vi "Sequence.GetiStepProperties.vi"(7 "Iteration":string, 8 "error in (no error)":errorcluster, 11 "Elements":T1[](array[typedef])) -> (0 "error out":errorcluster, 1 "Step Conatins iStep?":bool, 3 "iStepForLoop Ref":refnum<k24>)   [LabVIEW 2013, in "Simple Sequence Tools - Editor.lvlib"]
uses:
  Simple Sequence Tools - Editor.lvlib
  Types/Compiled.StepElementProperties.ctl
  Shared/Types/Channel.Properties.ctl
  Shared/Types/Step.Types.ctl
  NationalInstruments.VeriStand.RealTimeSequenceDefinitionApi
  Shared/SubVIs/Main.Constants.vi
  Shared/Simple Sequence Tools - Shared.lvlib
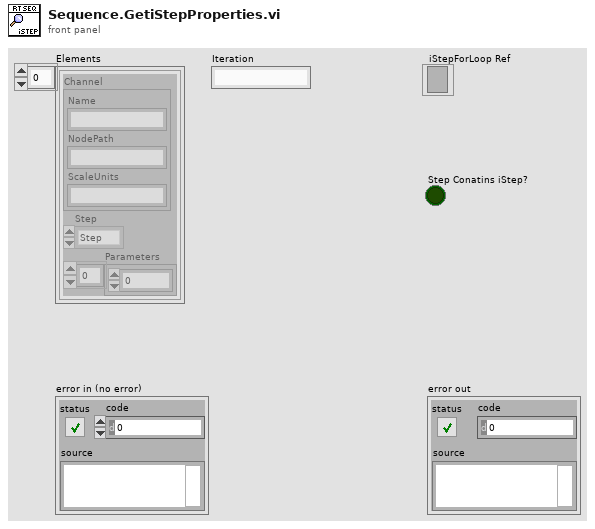
[diagram p1: front panel]
types:
  T1 = typedef "Simple Sequence Tools - Editor.lvlib/Compiled.StepElementProperties.ctl" = cluster{"Channel":T2, "Step":T3, "Parameters":dbl[]}
  T2 = typedef "Simple Sequence Tools - Shared.lvlib/Channel.Properties.ctl" = cluster{"Name":string, "NodePath":string, "ScaleUnits":string}
  T3 = typedef "Simple Sequence Tools - Shared.lvlib/Step.Types.ctl" = enum8{"Step", "iStep", "Ramp", "Unchanged", "Unknown", "Sine", "LogSine", "LinearSine", "ForcedRamp"}
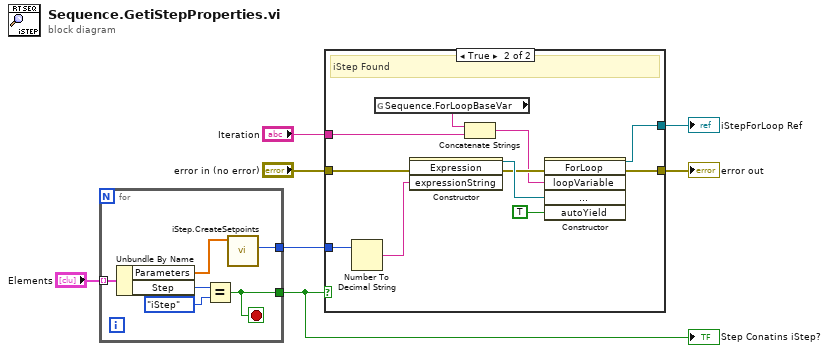
[diagram p0: block diagram]
diagram:
  n1 = for {
    tunnel: "Elements" -> [w13] mode=indexing
    tunnel: [w8] -> w5
    tunnel: [w10] -> w3
    stop <- w10 stop-if-true
    n2 = Unbundle By Name(w13) -> ("Parameters"=w9:dbl[], "Step"=w12:T3)
    n3 = Equal?(x=w12, y=Step.Types."iStep") -> (x = y?=w10:bool)
    n4 = call "iStep.CreateSetpoints.vi"("Parameters"=w9) -> ("samples"=w8:i32)  [unwired: 9 in, 1 out]
  }
  "Step Conatins iStep?" <- w3
  n5 = case shown="True" w3 {
    tunnel: "error in (no error)" -> [w14 w23]
    tunnel: [w14 w22] -> w6
    tunnel: w5 -> [_ w21]
    tunnel: [_ w19] -> w4
    tunnel: "Iteration" -> [_ w17]
    frame False {
      # "No iStep in step"
    }
    frame True {
      # "iStep Found"
      n6 = Number To Decimal String(number=w21) -> (decimal integer string=w20:string)  [unwired: 1 in]
      n7 = global read "Main.Constants.vi" "Sequence.ForLoopBaseVar"() -> (w15:string)
      n8 = constructor class="Expression"(error in=w23, "expressionString"=w20) -> (reference out=w25:refnum<k24>, error out=w24:errorcluster)  [unwired: 2 in, 2 out]
      n9 = Concatenate Strings(w15, w17) -> (w16:string)
      n10 = constructor class="ForLoop"(error in=w24, "loopVariable"=w16, "iterations"=w25, "autoYield"=TRUE) -> (reference out=w19:refnum<k24>, error out=w22:errorcluster)  [unwired: 2 in, 4 out]
    }
  }
  "error out" <- w6
  "iStepForLoop Ref" <- w4
